vi "Game.vi"(8 "file path":path, 10 "Difficulty":enum16{"Easy", "Medium", "Hard"}(ring)) -> (2 "Game state":enum16{"Easy", "med", "hard", "over"}(ring))   [LabVIEW 2021]
uses:
  type defs/Score.ctl
  type defs/WIn Score.ctl
  type defs/Time Remaining.ctl
  <vilib>/Utility/miscctls.llb/LVPointTypeDef.ctl
  <vilib>/Utility/miscctls.llb/LVPoint32TypeDef.ctl
  <vilib>/numeric/Random Number (Range) U64.vi
  <vilib>/numeric/sub_Random U32.vi
  <vilib>/Utility/file.llb/Write Delimited Spreadsheet (string).vi
panel:
  out "Score Chart":i32(graph)
  out "time":string
  in  "Stop 2":bool
  out "Num of Circles":i32
  out "Time Remaining":T1
  out "Stop":bool
  out "Win Score":T2
  out "Difficulty 2":enum16{"Easy", "Medium", "Hard"}(ring)
  out "Score":T3
  out "Wrong":cluster{"horizontal":i16, "vertical":i16}[](array[cluster])
  out "Correct":cluster{"horizontal":i16, "vertical":i16}[](array[cluster])
  out "Size":i16
  in  "picture":picture
  # "REFLEX TRAINING GAME"
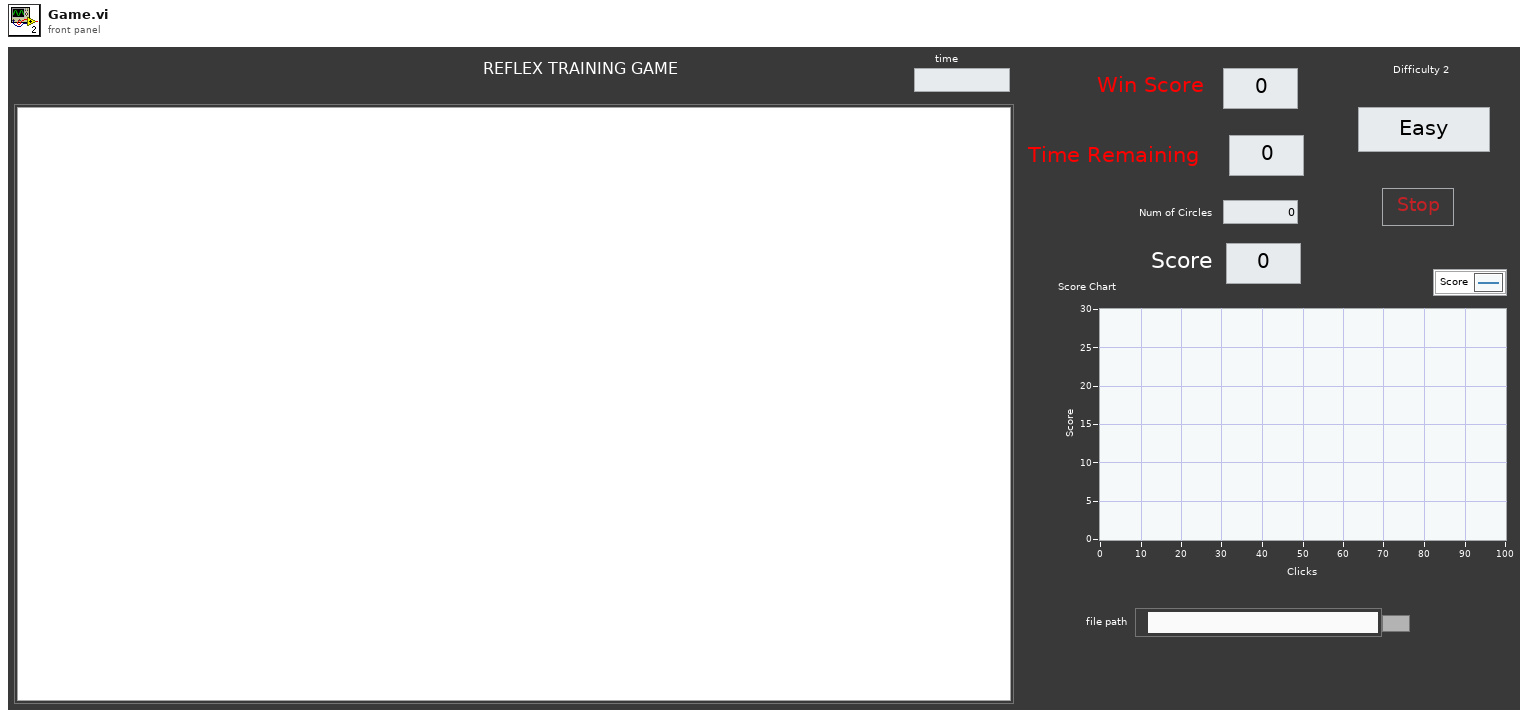
[diagram p1: front panel]
types:
  T1 = typedef "Time Remaining.ctl" = u8
  T2 = typedef "WIn Score.ctl" = i32
  T3 = typedef "Score.ctl" = i32
  T4 = typedef "LVPoint32TypeDef.ctl" = cluster{"Horizontal":i32, "Vertical":i32}
  T5 = typedef "LVPointTypeDef.ctl" = cluster{"Horizontal":i16, "Vertical":i16}
  T6 = typedef "LVPositionTypeDef.ctl" = cluster{"Left":i32, "Top":i32}
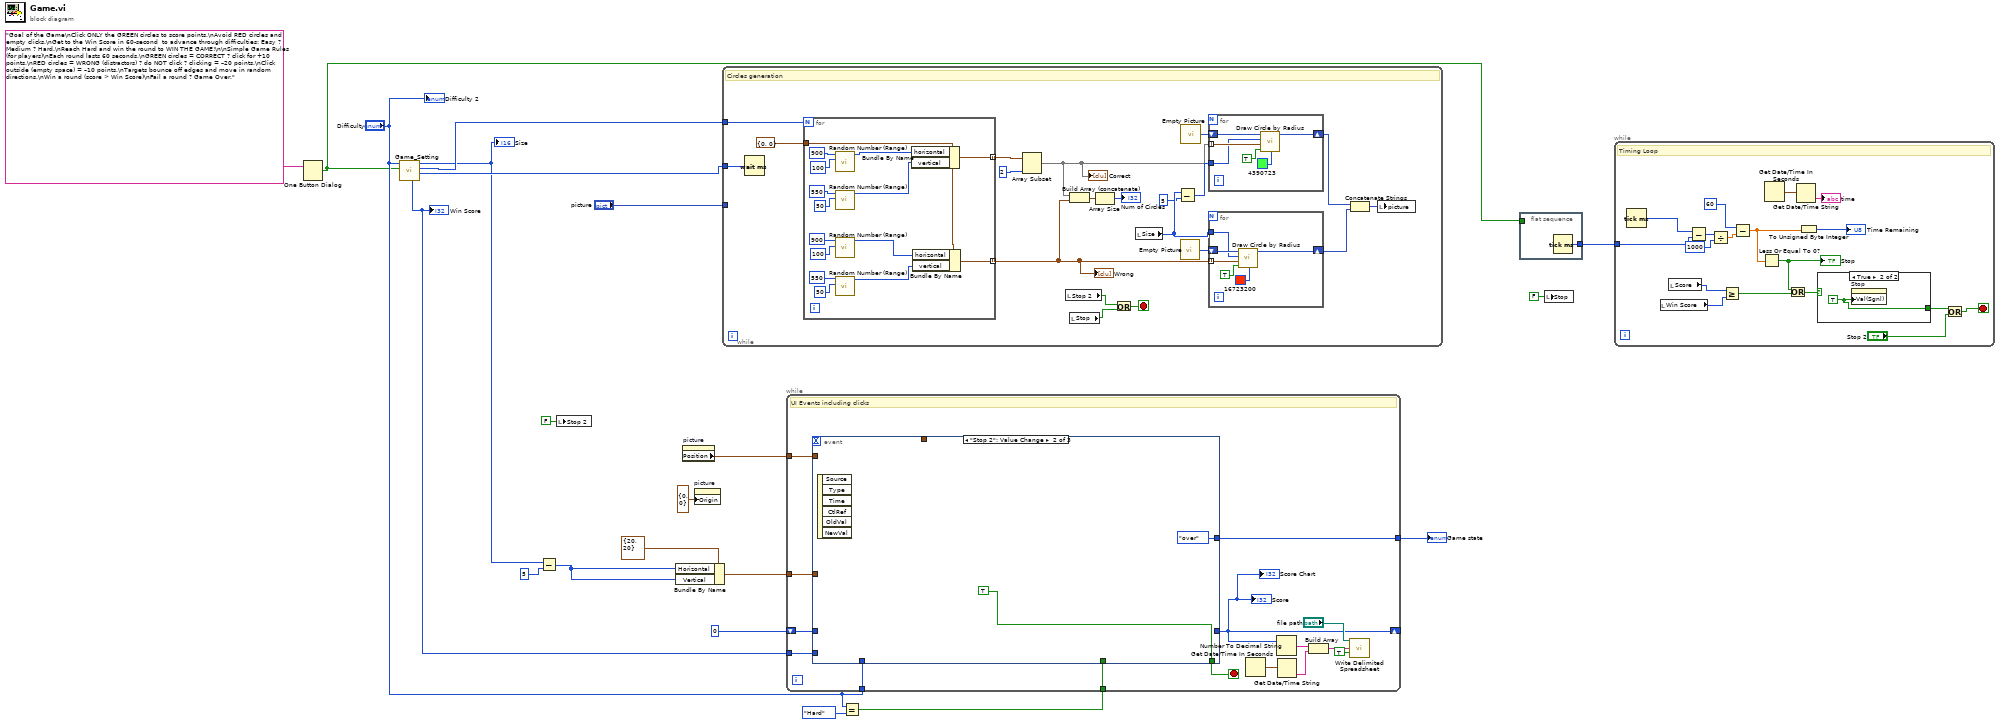
[diagram p0: block diagram]
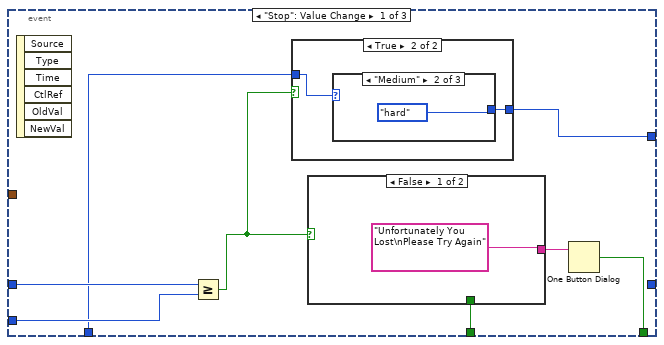
[diagram p3: hidden frame]
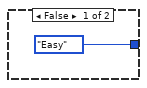
[diagram p4: hidden frame]
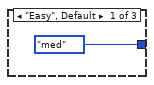
[diagram p5: hidden frame]
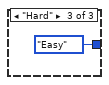
[diagram p6: hidden frame]
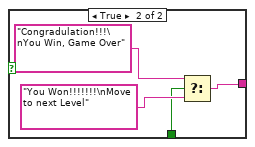
[diagram p7: hidden frame]
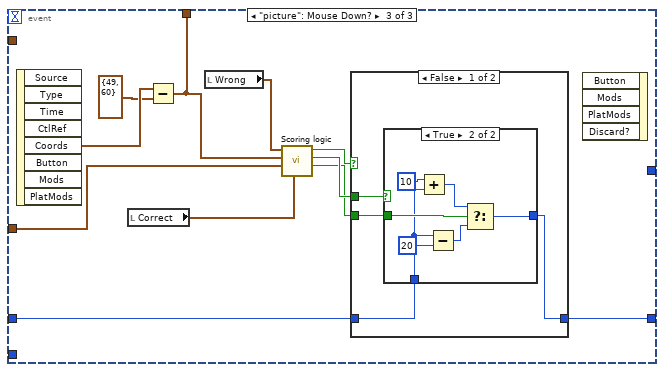
[diagram p8: hidden frame]
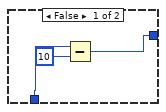
[diagram p9: hidden frame]
diagram:
  n1 = One Button Dialog(message="Goal of the Game\nClick ONLY the GREEN circles to score points.\nAvoid RED circles and empty clicks.\nGet to the Win Score in 60-second  to advance through difficulties: Easy ? Medium ? Hard.\nReach Hard and win the round to WIN THE GAME!\n\nSimple Game Rules (for players)\nEach round lasts 60 seconds.\nGREEN circles = CORRECT ? click for +10 points.\nRED circles = WRONG (distractors) ? do NOT click ? clicking = –20 points.\nClick outside (empty space) = –10 points.\nTargets bounce off edges and move in random directions.\nWin a round (score > Win Score)\nFail a round ? Game Over.") -> (true=w2:bool)  [unwired: 1 in]
  n2 = call "Game_Setting.vi"("true"=w2, "Difficulty"="Difficulty") -> ("milliseconds to wait"=w19:u32, "Num of Circles"=w20:i32, "radius 2"=w14:i16, "radius"=w9:i16)  [unwired: 6 in]
  "Size" <- w14
  "Win Score" <- w9
  n3 = Subtract(x=w14, y=i16 5 ("x")) -> (x-y=w12:i16)
  n4 = local write "Stop 2"(FALSE ("Stop 2")) -> ()
  n5 = Bundle By Name(cluster=T4 {"Horizontal"=20, "Vertical"=20} ("x"), "Horizontal"=w12, "Vertical"=w12) -> (w13:T4)
  n6 = property on="picture" class="Pict"() -> ("Position"=w16:T6)  [unwired: 2 in, 2 out]
  n7 = property on="picture" class="Pict"("Origin"=T5 {"Horizontal"=0, "Vertical"=0}) -> ()  [unwired: 2 in, 2 out]
  n8 = while {
    tunnel: "picture" -> [_]
    tunnel: w20 -> [w41]
    tunnel: w19 -> [w31]
    stop <- w23 stop-if-true
    # "Circles generation"
    n9 = Wait (ms)(milliseconds to wait=w31) -> ()  [unwired: 1 out]
    n10 = for {
      N: w41 -> [_]
      tunnel: cluster{"horizontal":i16, "vertical":i16} {"horizontal"=0, "vertical"=0} ("pixel center") -> [w54]
      tunnel: [w62] -> w36 mode=indexing
      tunnel: [w55] -> w29 mode=indexing
      n11 = call-poly <vilib>:"Random Number (Range).vi"("lower bound (0)"=u64 100, "upper bound (100)"=u64 900) -> ("number"=w64:u64)  [unwired: 9 in]
      n12 = call-poly <vilib>:"Random Number (Range).vi"("lower bound (0)"=u64 50, "upper bound (100)"=u64 550) -> ("number"=w63:u64)  [unwired: 9 in]
      n13 = call-poly <vilib>:"Random Number (Range).vi"("lower bound (0)"=u64 100, "upper bound (100)"=u64 900) -> ("number"=w57:u64)  [unwired: 9 in]
      n14 = call-poly <vilib>:"Random Number (Range).vi"("lower bound (0)"=u64 50, "upper bound (100)"=u64 550) -> ("number"=w56:u64)  [unwired: 9 in]
      n15 = Bundle By Name(cluster=w54, "horizontal"=w64, "vertical"=w63) -> (w62:cluster{"horizontal":i16, "vertical":i16})
      n16 = Bundle By Name(cluster=w54, "horizontal"=w57, "vertical"=w56) -> (w55:cluster{"horizontal":i16, "vertical":i16})
    }
    "Wrong" <- w29
    n17 = Array Subset(array=w36, length=2) -> (w28:cluster{"horizontal":i16, "vertical":i16}[])  [unwired: 1 in]
    "Correct" <- w28
    n18 = local read "Stop 2"() -> (w22:bool)
    n19 = Build Array (concatenate)(w28, w29) -> (w26:cluster{"horizontal":i16, "vertical":i16}[])
    n20 = local read "Stop"() -> (w24:bool)
    n21 = Array Size(array=w26) -> (size(s)=→"Num of Circles":i32)
    n22 = Or(x=w22, y=w24) -> (x .or. y?=w23:bool)
    n23 = local read "Size"() -> (w34:i16)
    n24 = Subtract(x=w34, y=i16 5 ("x")) -> (x-y=w30:i16)
    n25 = call "Empty Picture"() -> ("empty picture"=w39:picture)
    n26 = call "Empty Picture"() -> ("empty picture"=w33:picture)
    n27 = for {
      tunnel: w28 -> [w47] mode=indexing
      tunnel: w30 -> [w42]
      shift-right: [w44] -> w32
      shift-left: w33 -> [w45]
      n28 = call <vilib>:"Draw Circle by Radius.vi"("color(black)"=u32 4390723, "fill?(F)"=TRUE, "pixel center"=w47, "radius"=w42, "picture"=w45) -> ("new picture"=w44:picture)  [unwired: 6 in]
    }
    n29 = for {
      tunnel: w29 -> [w53] mode=indexing
      tunnel: w34 -> [w48]
      shift-right: [w50] -> w38
      shift-left: w39 -> [w51]
      n30 = call <vilib>:"Draw Circle by Radius.vi"("color(black)"=u32 16723200, "fill?(F)"=TRUE, "pixel center"=w53, "radius"=w48, "picture"=w51) -> ("new picture"=w50:picture)  [unwired: 6 in]
    }
    n31 = Concatenate Strings(w32, w38) -> (w37:picture)
    n32 = local write "picture"(w37) -> ()
  }
  n33 = Equal?(x="Difficulty", y=enum16{"Easy", "Medium", "Hard"}."Hard") -> (x = y?=w7:bool)
  n34 = while {
    shift-right: [w71] -> _
    shift-left: 0 -> [w83]
    tunnel: w16 -> [w82]
    tunnel: w13 -> [w81]
    tunnel: w9 -> [w79]
    tunnel: w7 -> [w78]
    tunnel: "Difficulty" -> [w77]
    tunnel: [w76] -> w4
    stop <- w80 stop-if-true
    # "UI Events including clicks"
    n35 = event shown="[1] \"Stop 2\": Value Change" {
      selector: _ -> [_ _ _]
      dyn-events: _ -> [_ _ _]
      timeout: _ -> [_ _ _]
      tunnel: w83 -> [w90 _ w112]
      tunnel: [_ _ w111] -> w71
      tunnel: w82 -> [_ _ _]
      tunnel: [_ _ w106] -> _
      tunnel: w81 -> [_ _ w105]
      tunnel: [w87 TRUE ("true") _] -> w80
      tunnel: w79 -> [w91 _ _]
      tunnel: w78 -> [w89 _ _]
      tunnel: w77 -> [w85 _ _]
      tunnel: [w84 enum16{"Easy", "med", "hard", "over"}."over" ("y") _] -> w76
      event "Stop": Value Change {
        n36 = event-data() -> ()  [unwired: 1 in, 6 out]
        n37 = Greater Or Equal?(x=w90, y=w91) -> (x >= y?=w86:bool)
        n38 = case shown="True" w86 {
          tunnel: w85 -> [_ w94]
          tunnel: [enum16{"Easy", "med", "hard", "over"}."Easy" ("y") w93] -> w84
          frame False {
          }
          frame True {
            n39 = case shown="\"Medium\"" w94 {
              tunnel: [enum16{"Easy", "med", "hard", "over"}."med" ("y") enum16{"Easy", "med", "hard", "over"}."hard" ("y") enum16{"Easy", "med", "hard", "over"}."Easy" ("y")] -> w93
              frame "Easy", Default {
              }
              frame "Medium" {
              }
              frame "Hard" {
              }
            }
          }
        }
        n40 = case shown="False" w86 {
          tunnel: w89 -> [_ w99]
          tunnel: ["Unfortunately You Lost\nPlease Try Again" ("message") w100] -> w88
          frame False {
          }
          frame True {
            n41 = Select(t="Congradulation!!!\nYou Win, Game Over" ("message"), s=w99, f="You Won!!!!!!!\nMove to next Level" ("message")) -> (s? t:f=w100:string)
          }
        }
        n42 = One Button Dialog(message=w88) -> (true=w87:bool)  [unwired: 1 in]
      }
      event "Stop 2": Value Change {
        n43 = event-data() -> ()  [unwired: 1 in, 6 out]
      }
      event "picture": Mouse Down? {
        n44 = event-data() -> ("Coords"=w108:T4)  [unwired: 1 in, 7 out]
        n45 = local read "Correct"() -> (w115:cluster{"horizontal":i16, "vertical":i16}[])
        n46 = Subtract(x=w108, y=T4 {"Horizontal"=49, "Vertical"=60} ("x")) -> (x-y=w106:T4)
        n47 = local read "Wrong"() -> (w114:cluster{"horizontal":i16, "vertical":i16}[])
        n48 = call "Scoring logic.vi"("Correct"=w115, "x"=w105, "Coords"=w106, "Wrong"=w114) -> ("Checkbox"=w109:bool, "Checkbox 2"=w110:bool, "Checkbox 3"=w113:bool)  [unwired: 5 in]
        n49 = case shown="False" w113 {
          tunnel: w112 -> [w117 w130]
          tunnel: [w116 w130] -> w111
          tunnel: w110 -> [w119 _]
          tunnel: w109 -> [w118 _]
          frame False {
            n50 = case shown="True" w119 {
              tunnel: w118 -> [_ w129]
              tunnel: w117 -> [w122 w125]
              tunnel: [w120 w123] -> w116
              frame False {
                n51 = Subtract(x=w122, y=10) -> (x-y=w120:i32)
              }
              frame True {
                n52 = Add(x=10, y=w125) -> (x+y=w127:i32)
                n53 = Subtract(x=w125, y=20) -> (x-y=w126:i32)
                n54 = Select(t=w127, s=w129, f=w126) -> (s? t:f=w123:i32)
              }
            }
          }
          frame True {
          }
        }
        n55 = event-data() -> ()  [unwired: 5 in, 1 out]
      }
    }
    "Score" <- w71
    "Score Chart" <- w71
    n56 = Get Date/Time In Seconds() -> (seconds since 1Jan1904=w75:timestamp)
    n57 = Number To Decimal String(number=w71) -> (decimal integer string=w74:string)  [unwired: 1 in]
    n58 = Get Date/Time String(seconds (now)=w75) -> (time string=w69:string)  [unwired: 2 in, 1 out]
    n59 = Build Array(w74, w69) -> (w73:string[])
    n60 = call-poly <vilib>:"Write Delimited Spreadsheet.vi"("file path (dialog if empty)"="file path", "1D data"=w73, "append to file? (new file:F)"=TRUE) -> ()  [unwired: 11 in, 2 out]
  }
  "Game state" <- w4
  n61 = flat-sequence {
    tunnel: [w131] -> w10
    tunnel: w2 -> [_]
    frame #0 {
      n62 = Tick Count (ms)() -> (millisecond timer value=w131:u32)
    }
  }
  n63 = local write "Stop"(FALSE ("Stop")) -> ()
  n64 = while {
    tunnel: w10 -> [w148]
    stop <- w135 stop-if-true
    # "Timing Loop"
    n65 = Tick Count (ms)() -> (millisecond timer value=w149:u32)
    n66 = local read "Win Score"() -> (w139:T2)
    n67 = local read "Score"() -> (w140:T3)
    n68 = Subtract(x=w149, y=w148) -> (x-y=w147:u32)
    n69 = Divide(x=w147, y=u32 1000) -> (x/y=w144:dbl)
    n70 = Greater Or Equal?(x=w140, y=w139) -> (x >= y?=w137:bool)
    n71 = Subtract(x=u32 60, y=w144) -> (x-y=w142:dbl)
    n72 = Less Or Equal To 0?(x=w142) -> (x <= 0?=w138:bool)
    "Stop" <- w138
    n73 = Get Date/Time In Seconds() -> (seconds since 1Jan1904=w133:timestamp)
    n74 = Or(x=w138, y=w137) -> (x .or. y?=w136:bool)
    n75 = Get Date/Time String(seconds (now)=w133) -> (time string=→"time":string)  [unwired: 2 in, 1 out]
    n76 = To Unsigned Byte Integer(number=w142) -> (unsigned 8bit integer=→"Time Remaining":u8)
    n77 = case shown="True" w136 {
      selector: w136 -> [w150 _]
      tunnel: [w150 w151] -> w145
      frame False {
      }
      frame True {
        w151 = TRUE
        n78 = property on="Stop" class="Bool (strict)"("Val(Sgnl)"=w151) -> ()  [unwired: 2 in, 2 out]
      }
    }
    n79 = Or(x=w145, y="Stop 2") -> (x .or. y?=w135:bool)
  }
  "Difficulty 2" <- "Difficulty"
